vi "Autonomous Independent.vi"() -> ()   [LabVIEW 2017]
doc: "This VI is called when autonomous begins, and will automatically be terminated when autonomous ends. You can carry out timed or sensor driven robot movement independently without needing to return to the caller."
uses:
  GitHub/FIRST-3958-Controls-Library/NavX/navX Library v2/navX Library v2.lvlib
  <vilib>/addons/control/pid/NI_PID_pid.lvlib
  <vilib>/addons/control/pid/pid.llb/PID (DBL).vi
  <vilib>/Rock Robotics/WPI/ThirdParty/Phoenix-LabVIEW/Motor Controller/Controls/CTRE_Phoenix_MotorControl_ControlMode.ctl
  <vilib>/Rock Robotics/WPI/ThirdParty/Phoenix-LabVIEW/Motor Controller/Get/CTRE_Phoenix_MotorController_GetSelectedSensorData.vi
  GitHub/FIRST-3958-Controls-Library/NavX/navX Library v2/TypeDefs/Z900_navX_ZeroVectorTypeDef.ctl
  <vilib>/Rock Robotics/Network Tables/NT Write Numeric Array.vi
  <vilib>/Rock Robotics/Network Tables/NT Read String.vi
panel:
  in  "Array":cluster{"Amount":dbl, "Type":string}[](array[cluster])
  out "Yaw":dbl
  out "FR Pos":i32
  out "RL Pos":i32
  out "RR Pos":i32
  out "FL Pos":i32
  out "Displacement Z":dbl
  out "Displacement Y":dbl
  out "Displacement X":dbl
  out "Left":dbl(graph)
  out "Right":dbl(graph)
  in  "PID gains":T1={"proportional gain (Kc)"=0.1, "integral time (Ti, min)"=0.0, "derivative time (Td, min)"=0.0} {"derivative time (Td, min)" format="%.3f"; "integral time (Ti, min)" format="%.3f"; "proportional gain (Kc)" format="%.3f"}
  in  "Angle PID":T1={"proportional gain (Kc)"=1.8, "integral time (Ti, min)"=0.0, "derivative time (Td, min)"=0.0} {"derivative time (Td, min)" format="%.3f"; "integral time (Ti, min)" format="%.3f"; "proportional gain (Kc)" format="%.3f"}
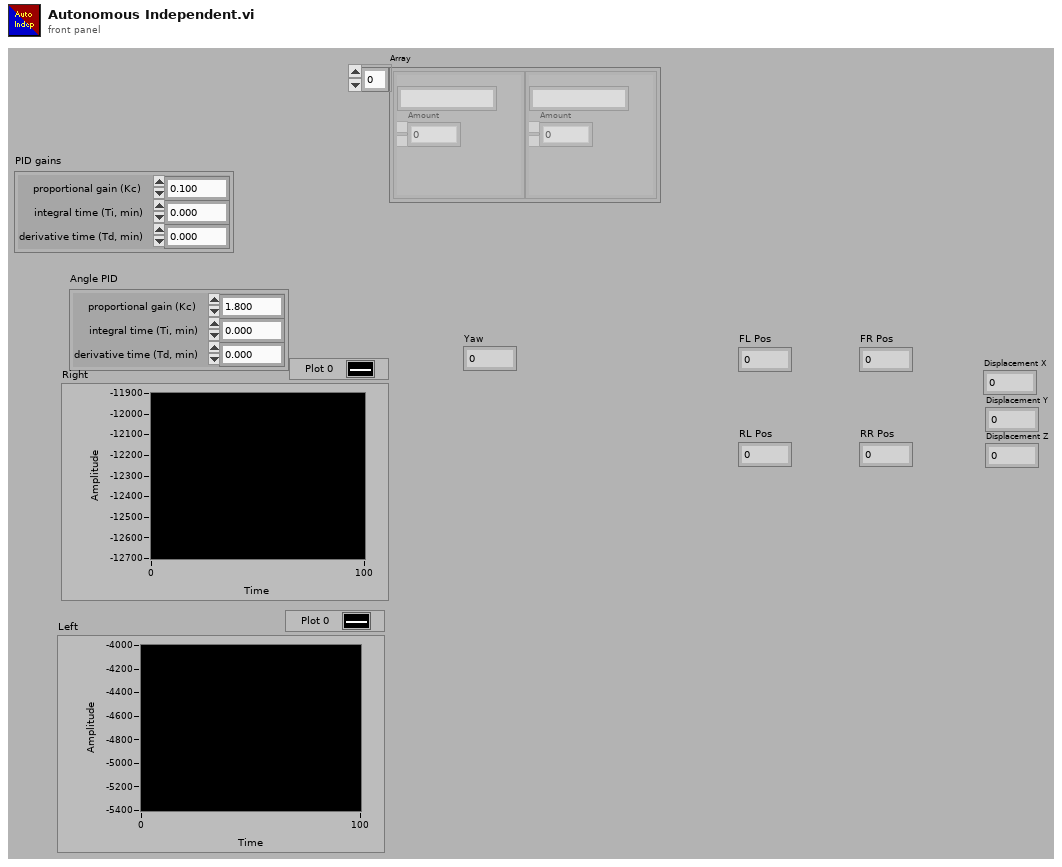
[diagram p1: front panel]
types:
  T1 = cluster{"proportional gain (Kc)":dbl, "integral time (Ti, min)":dbl, "derivative time (Td, min)":dbl}
  T2 = typedef "navX Library v2.lvlib/Z900_navX_ZeroVectorTypeDef.ctl" = cluster{"X":bool, "Y":bool, "Z":bool}
  T3 = typedef "WPI_JoystickDevRef.ctl" = cluster{"Device":T4}
  T4 = typedef "WPI_JoystickDeviceEnum.ctl" = enum16{"USB 0", "USB 1", "USB 2", "USB 3", "USB 4", "USB 5"}
  T5 = typedef "WPI_MotorControlDeviceRef.ctl" = cluster{"DeviceStatus":errorcluster, "Type":T6, "PWM":cluster{"PWM Channel":T7, "DeadBand":T8}, "CAN":cluster{"Device Number":u8, "SetOutput VI Ref":variant, "GetOutput VI Ref":variant, "Enable VI Ref":variant, "Disable VI Ref":variant, "Data":variant}, "Invert":bool, "DIO PWM":cluster{"PWM \"Enable\" Channel":T7, "DIOChannel":T9, "PWM Rate":dbl}}
  T6 = typedef "WPI_MotorControlType.ctl" = enum16{"PWM", "CAN", "DIO PWM"}
  T7 = typedef "FPGA_DIOPWMChannel.ctl" = enum8{"PWM 0", "PWM 1", "PWM 2", "PWM 3", "PWM 4", "PWM 5", "PWM 6", "PWM 7", "PWM 8", "PWM 9", "PWM MXP 0", "PWM MXP 1", "PWM MXP 2", "PWM MXP 3", "PWM MXP 4", "PWM MXP 5", "PWM MXP 6", "PWM MXP 7", "PWM MXP 8", "PWM MXP 9", "Invalid"}
  T8 = typedef "WPI_PWMDeadband.ctl" = cluster{"Name":string, "maxPositivePwm":i32, "minPositivePwm":i32, "centerPwm":i32, "maxNegativePwm":i32, "minNegativePwm":i32, "angularRange":u16}
  T9 = typedef "FPGA_DIOChannel.ctl" = enum8{"DIO 0", "DIO 1", "DIO 2", "DIO 3", "DIO 4", "DIO 5", "DIO 6", "DIO 7", "DIO 8", "DIO 9", "DIO MXP 0", "DIO MXP 1", "DIO MXP 2", "DIO MXP 3", "DIO MXP 4", "DIO MXP 5", "DIO MXP 6", "DIO MXP 7", "DIO MXP 8", "DIO MXP 9", "DIO MXP 10", "DIO MXP 11", "DIO MXP 12", "DIO MXP 13", "DIO MXP 14", "DIO MXP 15", "SPI Port CS1", "SPI Port CS2", "SPI Port CS3", "SPI Port MISO", "SPI Port MOSI", "Invalid"}
  T10 = typedef "navX Library v2.lvlib/Z900_navX_DeviceTypeDef.ctl" = cluster{"Interface":cluster{"Protocol":T11, "Update Rate (4Hz-100Hz)":u8, "navX Open TypeDef":variant}, "Notify Packet":refnum<notifier>, "Loop VI Refnum":refnum<vi>, "Ready to Close Occurrence Refnum":refnum<k4>}
  T11 = typedef "navX Library v2.lvlib/Z900_navX_ProtocolTypeDef.ctl" = enum16{"SERIAL", "I2C", "SPI"}
  T12 = typedef "CTRE_Phoenix_MotorControl_ControlMode.ctl" = u16
  T13 = cluster{"Yaw":dbl, "Roll":dbl, "Pitch":dbl, "Heading":dbl, "Fused Heading":dbl}
  T14 = cluster{"Velocity X":dbl, "Velocity Y":dbl, "Velocity Z":dbl, "Displacement X":dbl, "Displacement Y":dbl, "Displacement Z":dbl}
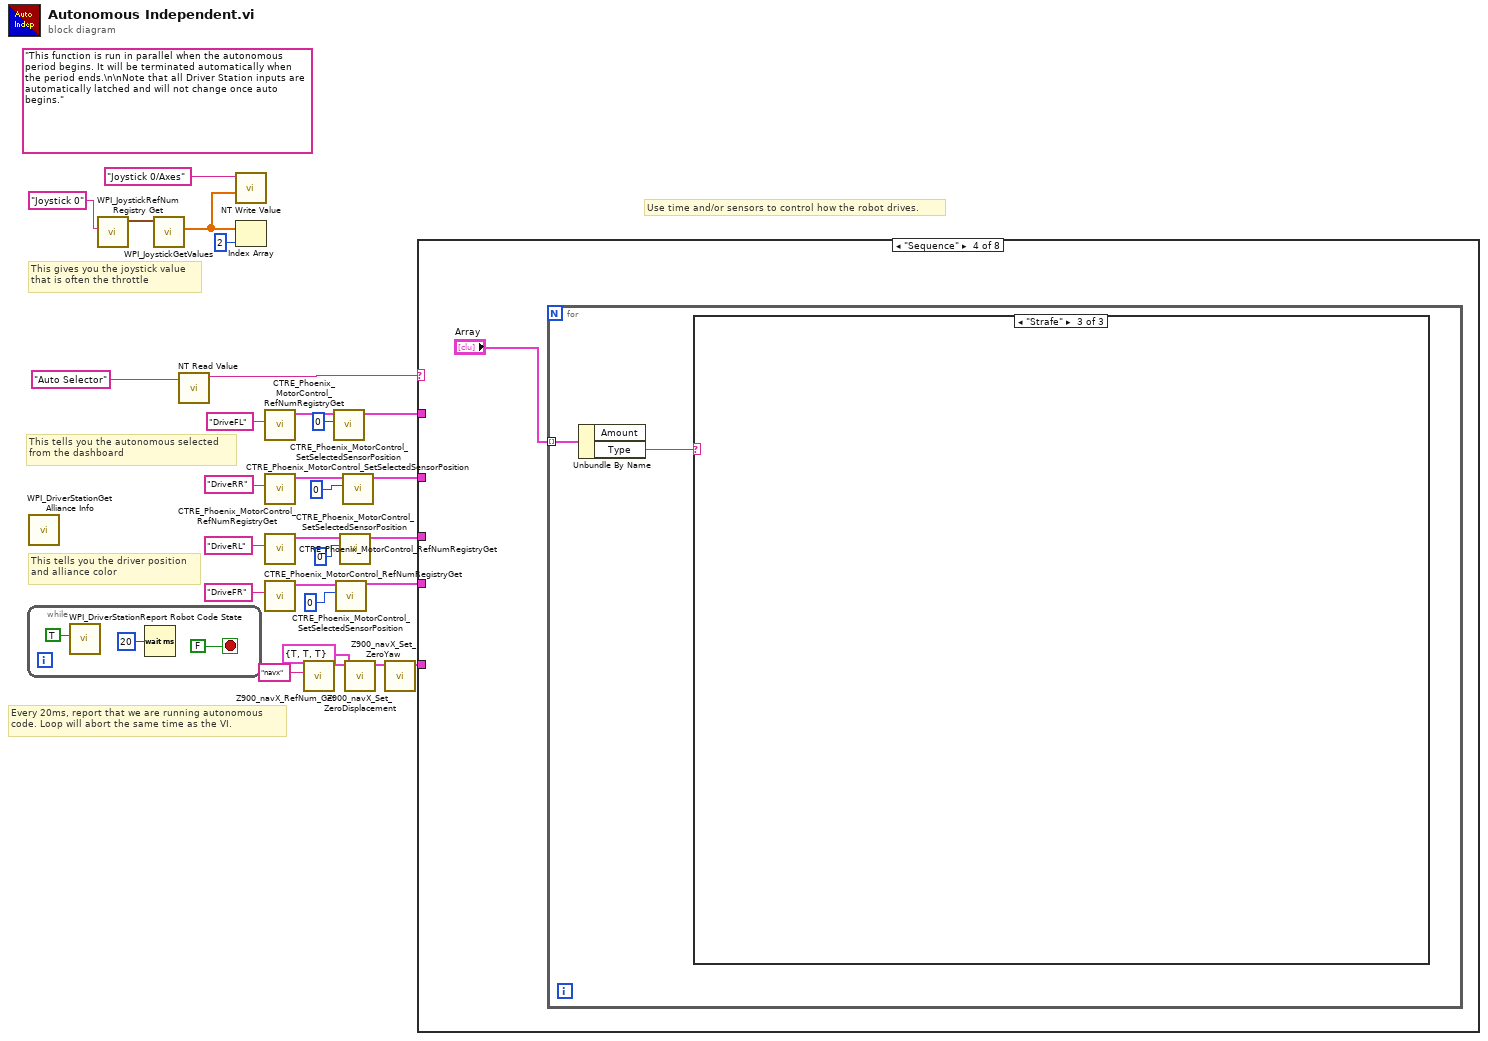
[diagram p0: block diagram]
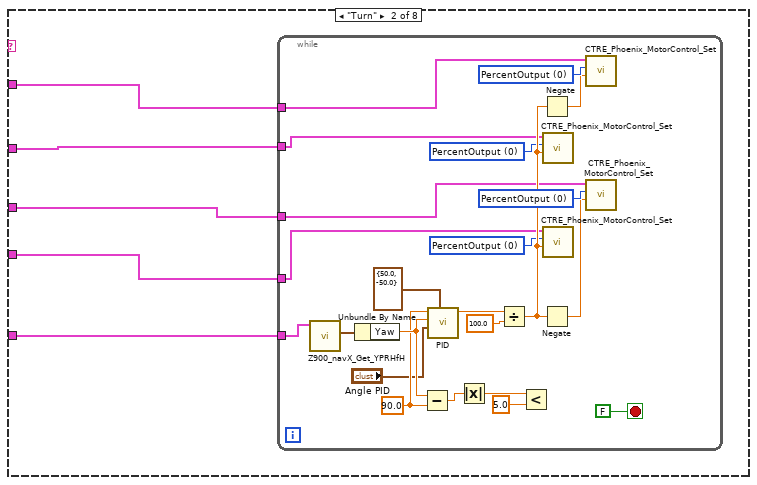
[diagram p3: hidden frame]
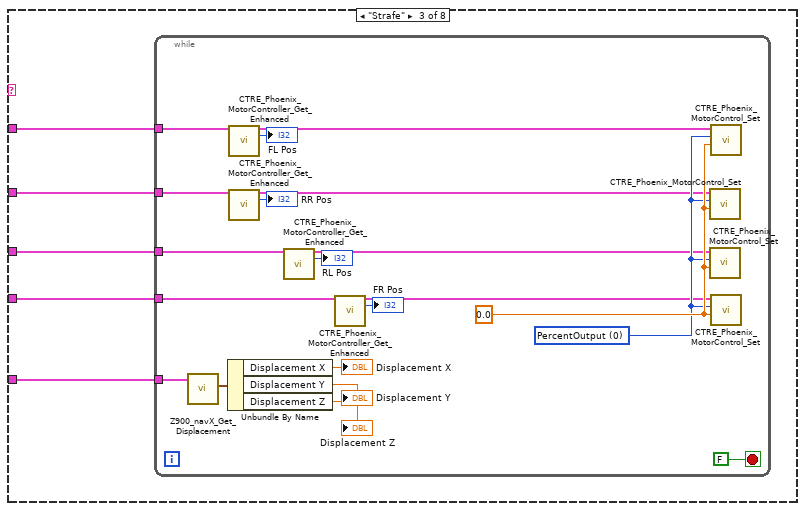
[diagram p4: hidden frame]
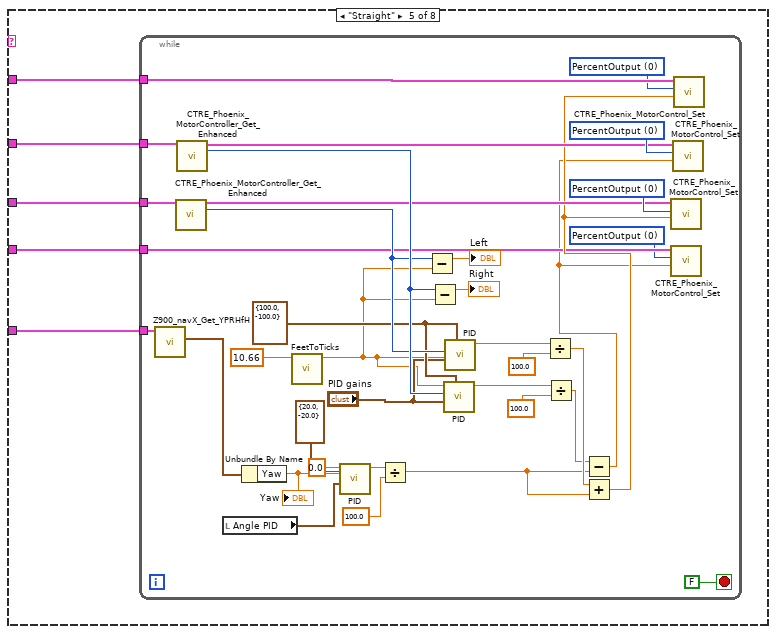
[diagram p7: hidden frame]
diagram:
  (unwired) "This function is run in parallel when the autonomous period begins. It will be terminated automatically when the period ends.\n\nNote that all Driver Station inputs are automatically latched and will not change once auto begins."
  # "This tells you the autonomous selected\nfrom the dashboard"
  # "Every 20ms, report that we are running autonomous\ncode. Loop will abort the same time as the VI."
  # "This gives you the joystick value\nthat is often the throttle"
  # "Use time and/or sensors to control how the robot drives."
  # "This tells you the driver position\nand alliance color"
  n1 = while {
    stop <- FALSE stop-if-true
    n2 = call <vilib>:"WPI_DriverStationReport Robot Code State.vi"("Autonomous"=TRUE) -> ()  [unwired: 10 in, 1 out]
    n3 = Wait (ms)(milliseconds to wait=u32 20) -> ()  [unwired: 1 out]
  }
  n4 = call <vilib>:"WPI_DriverStationGet Alliance Info.vi"() -> ()  [unwired: 12 out]
  n5 = call <vilib>:"WPI_JoystickRefNum Registry Get.vi"("refnum name"="Joystick 0") -> ("JoystickDevRef"=w27:T3)  [unwired: 1 in, 9 out]
  n6 = call <vilib>:"WPI_JoystickGetValues.vi"("JoystickDevRef"=w27) -> ("Axes"=w23:dbl[])  [unwired: 6 in, 4 out]
  n7 = call-poly <vilib>:"NT Read Value.vi"("Name"="Auto Selector") -> ("String"=w24:string)  [unwired: 9 in, 1 out]
  n8 = call-poly <vilib>:"NT Write Value.vi"("Numeric Array"=w23, "Name"="Joystick 0/Axes") -> ()  [unwired: 9 in, 1 out]
  n9 = Index Array(array=w23, index=2) -> ()  [unwired: 1 out]
  n10 = call <vilib>:"CTRE_Phoenix_MotorControl_RefNumRegistryGet.vi"("refnum name"="DriveFL") -> ("PhoenixMotorControlDevRef"=w15:T5)  [unwired: 9 in, 1 out]
  n11 = call <vilib>:"CTRE_Phoenix_MotorControl_RefNumRegistryGet.vi"("refnum name"="DriveRR") -> ("PhoenixMotorControlDevRef"=w17:T5)  [unwired: 9 in, 1 out]
  n12 = call <vilib>:"CTRE_Phoenix_MotorControl_RefNumRegistryGet.vi"("refnum name"="DriveRL") -> ("PhoenixMotorControlDevRef"=w11:T5)  [unwired: 9 in, 1 out]
  n13 = call <vilib>:"CTRE_Phoenix_MotorControl_RefNumRegistryGet.vi"("refnum name"="DriveFR") -> ("PhoenixMotorControlDevRef"=w16:T5)  [unwired: 9 in, 1 out]
  n14 = call "Z900_navX_RefNum_Get.vi"("refnum name"="navx") -> ("navX Device"=w3:T10)  [unwired: 9 in, 1 out]
  n15 = call <vilib>:"CTRE_Phoenix_MotorControl_SetSelectedSensorPosition.vi"("New Sensor Position"=0, "PhoenixMotorControlDevRef"=w15) -> ("PhoenixMotorControlDevRef"=w10:T5)  [unwired: 8 in, 1 out]
  n16 = call <vilib>:"CTRE_Phoenix_MotorControl_SetSelectedSensorPosition.vi"("New Sensor Position"=0, "PhoenixMotorControlDevRef"=w16) -> ("PhoenixMotorControlDevRef"=w9:T5)  [unwired: 8 in, 1 out]
  n17 = call <vilib>:"CTRE_Phoenix_MotorControl_SetSelectedSensorPosition.vi"("New Sensor Position"=0, "PhoenixMotorControlDevRef"=w11) -> ("PhoenixMotorControlDevRef"=w12:T5)  [unwired: 8 in, 1 out]
  n18 = call <vilib>:"CTRE_Phoenix_MotorControl_SetSelectedSensorPosition.vi"("New Sensor Position"=0, "PhoenixMotorControlDevRef"=w17) -> ("PhoenixMotorControlDevRef"=w14:T5)  [unwired: 8 in, 1 out]
  n19 = call "Z900_navX_Set_ZeroDisplacement.vi"("Zero Vector"=T2 {"X"=TRUE, "Y"=TRUE, "Z"=TRUE}, "navX Device"=w3) -> ("navX Device"=w2:T10)  [unwired: 8 in, 1 out]
  n20 = call "Z900_navX_Set_ZeroYaw.vi"("navX Device"=w2) -> ("navX Device"=w4:T10)  [unwired: 9 in, 1 out]
  n21 = case shown="\"Sequence\"" w24 {
    tunnel: w14 -> [_ w36 w63 _ w92 _ _ _]
    tunnel: w9 -> [_ w35 w61 _ w88 _ _ _]
    tunnel: w12 -> [_ w34 w62 _ w91 _ _ _]
    tunnel: w10 -> [_ w33 w64 _ w90 _ _ _]
    tunnel: w4 -> [_ w32 w60 _ w89 _ _ _]
    frame Default {
      # "You can put your main auto here, or you can right-click on the case and make any\nother frame be the default case."
      # "This is the frame that will execute if no selection is made, or if it is not recognized"
    }
    frame "Turn" {
      n22 = while {
        tunnel: w36 -> [w41]
        tunnel: w35 -> [w40]
        tunnel: w34 -> [w39]
        tunnel: w33 -> [w38]
        tunnel: w32 -> [w37]
        stop <- FALSE stop-if-true
        w49 = T12 0 items=["PercentOutput"=0, "Position"=1, "Velocity"=2, "Current"=3, "Follower"=5, "MotionProfile"=6, "MotionMagic"=7, "MotionMagicArc"=8, "MotionProfileArc"=10, "Disabled"=15] ("Control Mode")
        w50 = T12 0 items=["PercentOutput"=0, "Position"=1, "Velocity"=2, "Current"=3, "Follower"=5, "MotionProfile"=6, "MotionMagic"=7, "MotionMagicArc"=8, "MotionProfileArc"=10, "Disabled"=15] ("Control Mode")
        w51 = T12 0 items=["PercentOutput"=0, "Position"=1, "Velocity"=2, "Current"=3, "Follower"=5, "MotionProfile"=6, "MotionMagic"=7, "MotionMagicArc"=8, "MotionProfileArc"=10, "Disabled"=15] ("Control Mode")
        w52 = T12 0 items=["PercentOutput"=0, "Position"=1, "Velocity"=2, "Current"=3, "Follower"=5, "MotionProfile"=6, "MotionMagic"=7, "MotionMagicArc"=8, "MotionProfileArc"=10, "Disabled"=15] ("Control Mode")
        w57 = 90.0 ("setpoint")
        n23 = call "Z900_navX_Get_YPRHfH.vi"("navX Device"=w37) -> ("YRPHfH"=w59:T13)  [unwired: 7 in, 3 out]
        n24 = Unbundle By Name(w59) -> ("Yaw"=w58:dbl)
        n25 = Subtract(x=w58, y=w57) -> (x-y=w45:dbl)
        n26 = call-poly <vilib>:"PID.vi"("output range"=cluster{"output high":dbl, "output low":dbl} {"output high"=50.0, "output low"=-50.0}, "PID gains"="Angle PID", "process variable"=w58, "setpoint"=w57) -> ("output"=w55:dbl)  [unwired: 6 in, 1 out]
        n27 = Absolute Value(x=w45) -> (abs(x)=w44:dbl)
        n28 = Divide(x=w55, y=100.0) -> (x/y=w53:dbl)
        n29 = Less?(x=w44, y=5.0) -> ()  [unwired: 1 out]
        n30 = Negate(x=w53) -> (-x=w46:dbl)
        n31 = Negate(x=w53) -> (-x=w47:dbl)
        n32 = call <vilib>:"CTRE_Phoenix_MotorControl_Set.vi"("Output"=w53, "Control Mode"=w49, "PhoenixMotorControlDevRef"=w41) -> ()  [unwired: 7 in, 2 out]
        n33 = call <vilib>:"CTRE_Phoenix_MotorControl_Set.vi"("Output"=w53, "Control Mode"=w51, "PhoenixMotorControlDevRef"=w40) -> ()  [unwired: 7 in, 2 out]
        n34 = call <vilib>:"CTRE_Phoenix_MotorControl_Set.vi"("Output"=w46, "Control Mode"=w52, "PhoenixMotorControlDevRef"=w38) -> ()  [unwired: 7 in, 2 out]
        n35 = call <vilib>:"CTRE_Phoenix_MotorControl_Set.vi"("Output"=w47, "Control Mode"=w50, "PhoenixMotorControlDevRef"=w39) -> ()  [unwired: 7 in, 2 out]
      }
    }
    frame "Strafe" {
      n36 = while {
        tunnel: w64 -> [w76]
        tunnel: w63 -> [w74]
        tunnel: w62 -> [w72]
        tunnel: w61 -> [w70]
        tunnel: w60 -> [w84]
        stop <- FALSE stop-if-true
        w77 = T12 0 items=["PercentOutput"=0, "Position"=1, "Velocity"=2, "Current"=3, "Follower"=5, "MotionProfile"=6, "MotionMagic"=7, "MotionMagicArc"=8, "MotionProfileArc"=10, "Disabled"=15] ("Control Mode")
        w79 = 0.0 ("Output")
        n37 = call "Z900_navX_Get_Displacement.vi"("navX Device"=w84) -> ("Displacement"=w83:T14)  [unwired: 7 in, 3 out]
        n38 = Unbundle By Name(w83) -> ("Displacement X"=→"Displacement X":dbl, "Displacement Y"=→"Displacement Y":dbl, "Displacement Z"=→"Displacement Z":dbl)
        n39 = call-poly <vilib>:"CTRE_Phoenix_MotorController_Get_Enhanced.vi"("PhoenixMotorControlDevRef"=w76) -> ("PhoenixMotorControlDevRef"=w75:T5, "Position (Raw Sensor Units)"=→"FL Pos":i32)  [unwired: 11 in, 2 out]
        n40 = call-poly <vilib>:"CTRE_Phoenix_MotorController_Get_Enhanced.vi"("PhoenixMotorControlDevRef"=w74) -> ("PhoenixMotorControlDevRef"=w73:T5, "Position (Raw Sensor Units)"=→"RR Pos":i32)  [unwired: 11 in, 2 out]
        n41 = call-poly <vilib>:"CTRE_Phoenix_MotorController_Get_Enhanced.vi"("PhoenixMotorControlDevRef"=w72) -> ("PhoenixMotorControlDevRef"=w71:T5, "Position (Raw Sensor Units)"=→"RL Pos":i32)  [unwired: 11 in, 2 out]
        n42 = call-poly <vilib>:"CTRE_Phoenix_MotorController_Get_Enhanced.vi"("PhoenixMotorControlDevRef"=w70) -> ("PhoenixMotorControlDevRef"=w69:T5, "Position (Raw Sensor Units)"=→"FR Pos":i32)  [unwired: 11 in, 2 out]
        n43 = call <vilib>:"CTRE_Phoenix_MotorControl_Set.vi"("Output"=w79, "Control Mode"=w77, "PhoenixMotorControlDevRef"=w73) -> ()  [unwired: 7 in, 2 out]
        n44 = call <vilib>:"CTRE_Phoenix_MotorControl_Set.vi"("Output"=w79, "Control Mode"=w77, "PhoenixMotorControlDevRef"=w71) -> ()  [unwired: 7 in, 2 out]
        n45 = call <vilib>:"CTRE_Phoenix_MotorControl_Set.vi"("Output"=w79, "Control Mode"=w77, "PhoenixMotorControlDevRef"=w75) -> ()  [unwired: 7 in, 2 out]
        n46 = call <vilib>:"CTRE_Phoenix_MotorControl_Set.vi"("Output"=w79, "Control Mode"=w77, "PhoenixMotorControlDevRef"=w69) -> ()  [unwired: 7 in, 2 out]
      }
    }
    frame "Sequence" {
      n47 = for {
        tunnel: "Array" -> [w87] mode=indexing
        n48 = Unbundle By Name(w87) -> ("Type"=w86:string)  [unwired: 1 out]
        n49 = case shown="\"Strafe\"" w86 {
          frame "Turn" {
          }
          frame "Straight" {
          }
          frame "Strafe" {
          }
        }
      }
    }
    frame "Straight" {
      n50 = while {
        tunnel: w92 -> [w128]
        tunnel: w91 -> [w127]
        tunnel: w90 -> [w119]
        tunnel: w89 -> [w117]
        tunnel: w88 -> [w102]
        stop <- FALSE stop-if-true
        w118 = T12 0 items=["PercentOutput"=0, "Position"=1, "Velocity"=2, "Current"=3, "Follower"=5, "MotionProfile"=6, "MotionMagic"=7, "MotionMagicArc"=8, "MotionProfileArc"=10, "Disabled"=15] ("Control Mode")
        w101 = T12 0 items=["PercentOutput"=0, "Position"=1, "Velocity"=2, "Current"=3, "Follower"=5, "MotionProfile"=6, "MotionMagic"=7, "MotionMagicArc"=8, "MotionProfileArc"=10, "Disabled"=15] ("Control Mode")
        w122 = T12 0 items=["PercentOutput"=0, "Position"=1, "Velocity"=2, "Current"=3, "Follower"=5, "MotionProfile"=6, "MotionMagic"=7, "MotionMagicArc"=8, "MotionProfileArc"=10, "Disabled"=15] ("Control Mode")
        w123 = T12 0 items=["PercentOutput"=0, "Position"=1, "Velocity"=2, "Current"=3, "Follower"=5, "MotionProfile"=6, "MotionMagic"=7, "MotionMagicArc"=8, "MotionProfileArc"=10, "Disabled"=15] ("Control Mode")
        w124 = cluster{"output high":dbl, "output low":dbl} {"output high"=100.0, "output low"=-100.0} ("output range")
        n51 = call "Z900_navX_Get_YPRHfH.vi"("navX Device"=w117) -> ("YRPHfH"=w116:T13)  [unwired: 7 in, 3 out]
        n52 = call-poly <vilib>:"CTRE_Phoenix_MotorController_Get_Enhanced.vi"("PhoenixMotorControlDevRef"=w127) -> ("PhoenixMotorControlDevRef"=w120:T5, "Position (Raw Sensor Units)"=w125:i32)  [unwired: 11 in, 2 out]
        n53 = call-poly <vilib>:"CTRE_Phoenix_MotorController_Get_Enhanced.vi"("PhoenixMotorControlDevRef"=w128) -> ("PhoenixMotorControlDevRef"=w121:T5, "Position (Raw Sensor Units)"=w126:i32)  [unwired: 11 in, 2 out]
        n54 = local read "Angle PID"() -> (w110:T1)
        n55 = Unbundle By Name(w116) -> ("Yaw"=w115:dbl)
        "Yaw" <- w115
        n56 = call "FeetToTicks.vi"("x"=10.66) -> ("Numeric"=w95:dbl)  [unwired: 10 in]
        n57 = call-poly <vilib>:"PID.vi"("output range"=cluster{"output high":dbl, "output low":dbl} {"output high"=20.0, "output low"=-20.0}, "PID gains"=w110, "process variable"=w115, "setpoint"=0.0) -> ("output"=w112:dbl)  [unwired: 6 in, 1 out]
        n58 = Divide(x=w112, y=100.0) -> (x/y=w93:dbl)
        n59 = Subtract(x=w125, y=w95) -> (x-y=→"Left":dbl)
        n60 = Subtract(x=w126, y=w95) -> (x-y=→"Right":dbl)
        n61 = call-poly <vilib>:"PID.vi"("output range"=w124, "PID gains"="PID gains", "process variable"=w126, "setpoint"=w95) -> ("output"=w107:dbl)  [unwired: 6 in, 1 out]
        n62 = call-poly <vilib>:"PID.vi"("output range"=w124, "PID gains"="PID gains", "process variable"=w125, "setpoint"=w95) -> ("output"=w106:dbl)  [unwired: 6 in, 1 out]
        n63 = Divide(x=w106, y=100.0) -> (x/y=w105:dbl)
        n64 = Divide(x=w107, y=100.0) -> (x/y=w104:dbl)
        n65 = Subtract(x=w104, y=w93) -> (x-y=w100:dbl)
        n66 = Add(x=w105, y=w93) -> (x+y=w103:dbl)
        n67 = call <vilib>:"CTRE_Phoenix_MotorControl_Set.vi"("Output"=w103, "Control Mode"=w123, "PhoenixMotorControlDevRef"=w120) -> ()  [unwired: 7 in, 2 out]
        n68 = call <vilib>:"CTRE_Phoenix_MotorControl_Set.vi"("Output"=w100, "Control Mode"=w101, "PhoenixMotorControlDevRef"=w102) -> ()  [unwired: 7 in, 2 out]
        n69 = call <vilib>:"CTRE_Phoenix_MotorControl_Set.vi"("Output"=w100, "Control Mode"=w122, "PhoenixMotorControlDevRef"=w121) -> ()  [unwired: 7 in, 2 out]
        n70 = call <vilib>:"CTRE_Phoenix_MotorControl_Set.vi"("Output"=w103, "Control Mode"=w118, "PhoenixMotorControlDevRef"=w119) -> ()  [unwired: 7 in, 2 out]
      }
    }
    frame "Alternative 1" {
      # "This sample code describes robot movements in an array. You can extend it to control other motors\non your robot. You can also use file I/O to move the data to a text file."
    }
    frame "Alternative 2" {
    }
    frame "Your Turn" {
    }
  }
